vi "Aquire Data.vi"(8 "error in (no error)":errorcluster, 10 "Aqusition Time (s)":dbl, 11 "DAQ Controller in":refnum<class "DAQ Controller.lvclass">) -> (0 "error out":errorcluster, 3 "DAQ Controller out":refnum<class "DAQ Controller.lvclass">)   [LabVIEW 2022 SP3, in "DAQ Controller.lvclass"]
uses:
  DAQ Controller.lvclass
  DAQ Controller.lvclass/DAQ Controller.ctl
  XY Stage/Process Actor/Process Framework/Process State Data/Process State Data.lvclass/Process State Data.ctl
  DAQ Actor/DAQ Process Messages/Aquire Data Msg/Aquire Data Msg.lvclass/Aquire Data Msg.ctl
  XY Stage/Process Actor/Process Framework/Process State Data/Accessor/Write Abort.vi
  DAQ Actor/DAQ Process Messages/Aquire Data Msg/Aquire Data Msg.lvclass
  C:/Program Files/National Instruments/LabVIEW 2022/vi.lib/ActorFramework/Message/Message.lvclass
  XY Stage/Process Actor/Process Framework/Interlock Q Class/Interlock Q Class.lvclass
  XY Stage/Process Actor/Process Framework/Process State Data/Process State Data.lvclass
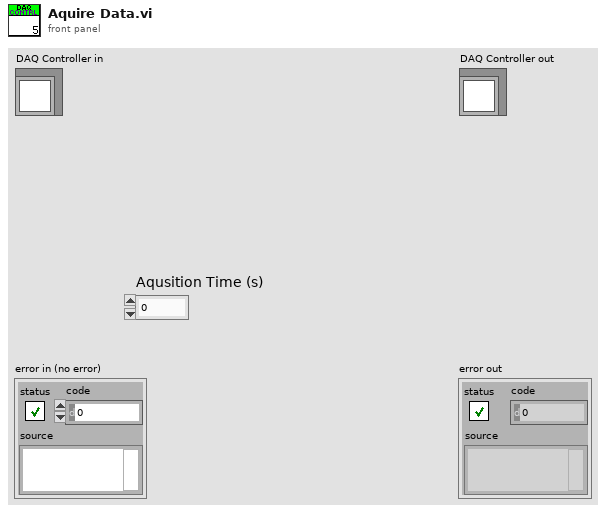
[diagram p1: front panel]
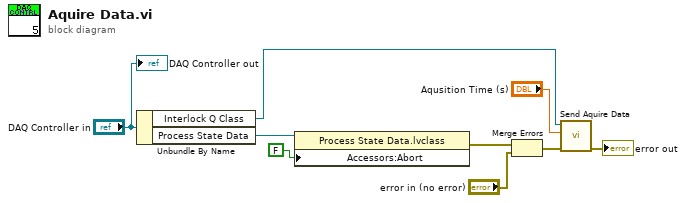
[diagram p0: block diagram]
diagram:
  n1 = Unbundle By Name("DAQ Controller in") -> ("Interlock Q Class"=w8:refnum<class "Interlock Q Class.lvclass">, "Process State Data"=w4:refnum<data-value>)
  n2 = property class="Process State Data.lvclass"(reference=w4, "Accessors:Abort"=FALSE ("Abort")) -> (error out=w1:errorcluster)  [unwired: 1 in, 1 out]
  n3 = Merge Errors(w1, "error in (no error)") -> (w2:errorcluster)
  n4 = call "Send Aquire Data.vi"("error in (no error)"=w2, "Aqusition Time (s)"="Aqusition Time (s)", "Interlock Q Class in"=w8) -> ("error out"=→"error out":errorcluster)  [unwired: 7 in, 1 out]
  "DAQ Controller out" <- "DAQ Controller in"
